vi "Write DedicatedEnQrs.vi"(10 "DedicatedEnQrs":refnum<queue>, 11 "CO2 Actor in":refnum<class "CO2 Actor.lvclass">) -> (3 "CO2 Actor out":refnum<class "CO2 Actor.lvclass">)   [LabVIEW 2015, in "cRIO-Carbondioxide.lvlib" / "CO2-Actor.lvlib" / "CO2 Actor.lvclass"]
uses:
  CO2 Actor.lvclass
  Controls/Dedicated Enqueuers.ctl
  <vilib>/ActorFramework/Message Enqueuer/Message Enqueuer.lvclass
  CO2 Actor.lvclass/CO2 Actor.ctl
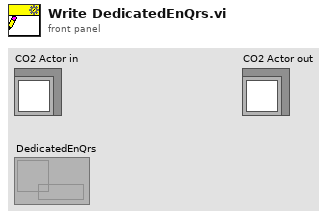
[diagram p1: front panel]
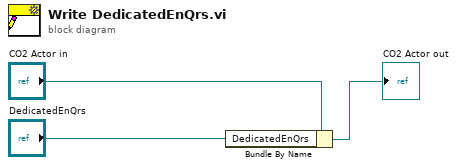
[diagram p0: block diagram]
diagram:
  n1 = Bundle By Name(cluster="CO2 Actor in", "DedicatedEnQrs"="DedicatedEnQrs") -> (→"CO2 Actor out":refnum<class "CO2 Actor.lvclass">)
